vi "FTW-Scheduler-GetNextJob.vi"(8 "error in":errorcluster, 10 "Jobs Performed":i32, 11 "FTW Job Scheduler":refnum<class "FTW-Scheduler.lvclass">) -> (0 "error out":errorcluster, 1 "Job Data":string, 2 "Current Job":string, 3 "FTW Job Scheduler out":refnum<class "FTW-Scheduler.lvclass">)   [LabVIEW 2015, in "FTW-Scheduler.lvclass"]
uses:
  FTW-Scheduler.lvclass
  FTW-Scheduler.lvclass/FTW-Scheduler.ctl
panel:
  # "Inputs"
  # "Outputs"
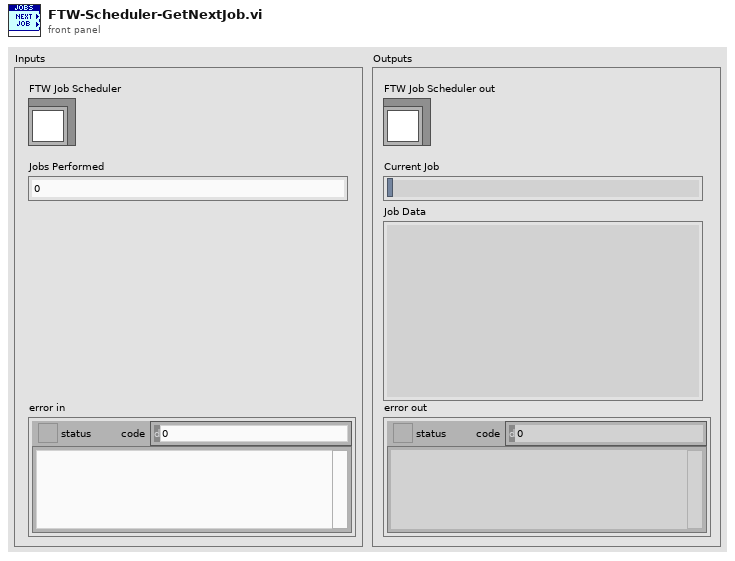
[diagram p1: front panel]
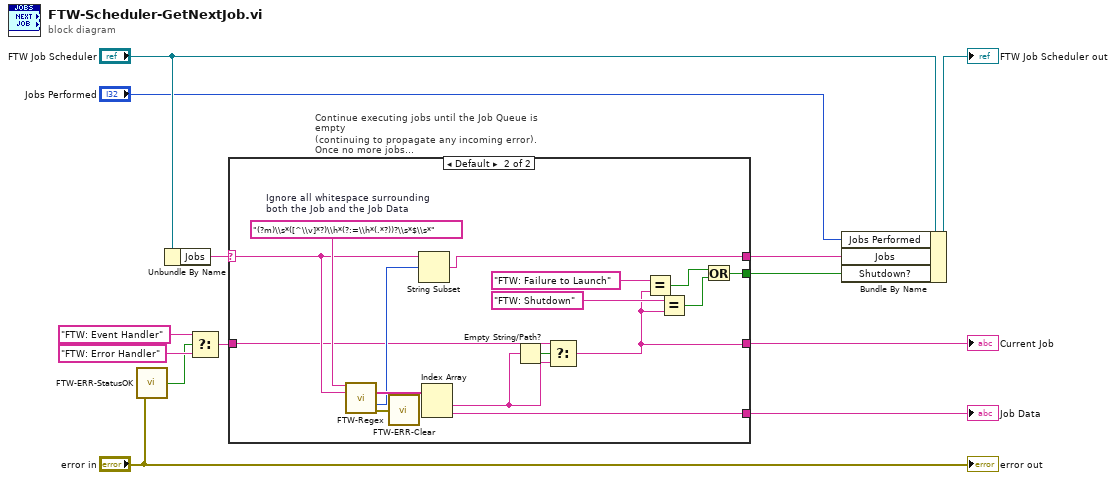
[diagram p0: block diagram]
diagram:
  n1 = call "FTW-ERR-StatusOK.vi"("error to check"="error in") -> ("Status OK?"=w5:bool)
  n2 = Unbundle By Name("FTW Job Scheduler") -> ("Jobs"=w2:string)
  n3 = Select(t="FTW: Event Handler", s=w5, f="FTW: Error Handler") -> (s? t:f=w4:string)
  n4 = case "Continue executing jobs until the Job Queue is empty\n(continuing to propagate any incoming error). Once no more jobs\nremain, handle error if exists; else, handle incoming inbox events." shown="Default" w2 {
    selector: w2 -> [w15 w25]
    tunnel: [w14 w19] -> w9
    tunnel: [_ w29] -> w12
    tunnel: [w15 w27] -> w3
    tunnel: [_ w17] -> w1
    tunnel: w4 -> [w14 w22]
    frame "" {
    }
    frame Default {
      w31 = "(?m)\\s*([^\\v]*?)\\h*(?:=\\h*(.*?))?\\s*$\\s*"  # Ignore all whitespace surrounding both the Job and the Job Data
      n5 = call "FTW-Regex.vi"("Regular Expression"=w31, "Input String"=w25) -> ("Submatches"=w30:string[], "Offset after Match"=w28:i32, "error out"=w26:errorcluster)  [unwired: 9 in, 2 out]
      n6 = call "FTW-ERR-Clear.vi"("error to snuff"=w26) -> ()  [unwired: 1 out]
      n7 = String Subset(string=w25, offset (0)=w28) -> (substring=w27:string)  [unwired: 1 in]
      n8 = Index Array(array=w30) -> (element #1=w21:string, element #2=w29:string)  [unwired: 2 in]
      n9 = Empty String/Path?(string/path=w21) -> (empty?=w23:bool)
      n10 = Select(t=w22, s=w23, f=w21) -> (s? t:f=w19:string)
      n11 = Equal?(x="FTW: Failure to Launch", y=w19) -> (x = y?=w16:bool)
      n12 = Equal?(x="FTW: Shutdown", y=w19) -> (x = y?=w18:bool)
      n13 = Or(x=w16, y=w18) -> (x .or. y?=w17:bool)
    }
  }
  "Current Job" <- w9
  "Job Data" <- w12
  n14 = Bundle By Name(cluster="FTW Job Scheduler", "Jobs Performed"="Jobs Performed", "Jobs"=w3, "Shutdown?"=w1) -> (→"FTW Job Scheduler out":refnum<class "FTW-Scheduler.lvclass">)
  "error out" <- "error in"
